vi "Begin.vi"() -> (0 "error out":errorcluster)   [LabVIEW 2013]
doc: "Called before other user functions, this VI is expected to open initial I/O refnums, load in file data, and do all program initialization. Notice that the <B>error out</B> terminal is simply used for data flow. Wiring it to other structures or subVIs ensures that this VI runs first."
uses:
  <vilib>/Rock Robotics/WPI/SafetyOutput/WPI_SafetyOutputConfigMenu.ctl
  <vilib>/Rock Robotics/WPI/DriverStation/WPI_DriverStationRobotMode2.ctl
  <vilib>/Rock Robotics/SystemInterfaces/DIO/FPGA_DIOPWMChannel.ctl
  <vilib>/Rock Robotics/SystemInterfaces/AI/FPGA_AIGyroChannel.ctl
  <vilib>/Rock Robotics/SystemInterfaces/Typedef/FPGA_TypedefAnalogModuleForGyro.ctl
  <vilib>/Rock Robotics/SystemInterfaces/DIO/FPGA_DIORelayChannel.ctl
  <vilib>/Rock Robotics/WPI/Joystick/WPI_JoystickDeviceEnum.ctl
  <vilib>/Rock Robotics/SystemInterfaces/DIO/FPGA_DIOChannel.ctl
  <vilib>/Rock Robotics/WPI/Encoder/WPI_EncoderType.ctl
  <vilib>/Rock Robotics/WPI/Relay/WPI_RelayDirection.ctl
  <vilib>/Rock Robotics/SystemInterfaces/Typedef/FPGA_TypedefDigitalModule.ctl
  <vilib>/Rock Robotics/WPI/Relay/WPI_RelayValue.ctl
  Robot Global Data.vi
  <vilib>/Rock Robotics/WPI/Counter/WPI_CounterDigitalInputToDigitalSource.vi
  <vilib>/Rock Robotics/WPI/MotorControl/WPI_MotorControlOpen Victor.vi
  <vilib>/Rock Robotics/WPI/RobotDrive/WPI_RobotDriveOpen4MotorWithVictor.vi
  <vilib>/Rock Robotics/WPI/Compressor/WPI_CompressorGetSetRefNum.vi
panel:
  out "error out 7":errorcluster
  out "error out 6":errorcluster
  out "error out 5":errorcluster
  out "error out 4":errorcluster
  out "error out 3":errorcluster
  out "error out 2":errorcluster
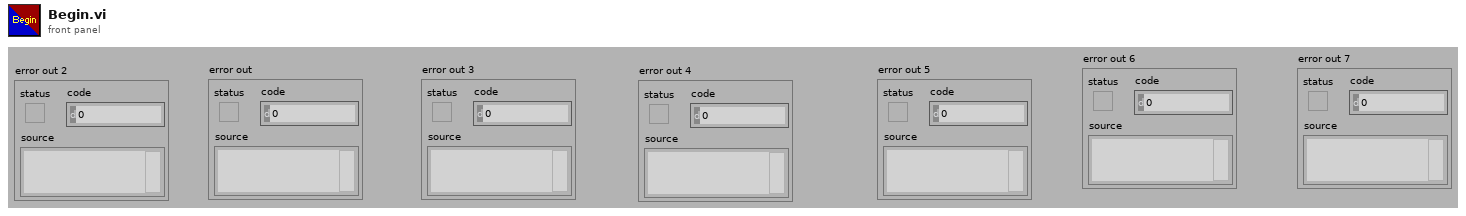
[diagram p1: front panel]
types:
  T1 = typedef "FPGA_DIOPWMChannel.ctl" = enum8{"PWM 1", "PWM 2", "PWM 3", "PWM 4", "PWM 5", "PWM 6", "PWM 7", "PWM 8", "PWM 9", "PWM 10", "Invalid"}
  T2 = typedef "WPI_RelayValue.ctl" = enum16{"Off", "On", "Forward", "Reverse"}
  T3 = typedef "FPGA_TypedefDigitalModule.ctl" = enum16{"Digital Module 1", "Digital Module 2"}
  T4 = typedef "FPGA_DIOChannel.ctl" = enum8{"DIO 1", "DIO 2", "DIO 3", "DIO 4", "DIO 5", "DIO 6", "DIO 7", "DIO 8", "DIO 9", "DIO 10", "DIO 11", "DIO 12", "DIO 13", "DIO 14", "Invalid"}
  T5 = typedef "FPGA_DIORelayChannel.ctl" = enum8{"Relay 1", "Relay 2", "Relay 3", "Relay 4", "Relay 5", "Relay 6", "Relay 7", "Relay 8", "Invalid"}
  T6 = typedef "WPI_RelayDirection.ctl" = enum16{"Both directions", "Forward only", "Reverse only"}
  T7 = typedef "WPI_EncoderType.ctl" = enum16{"1x", "2x", "4x"}
  T8 = typedef "WPI_JoystickDeviceEnum.ctl" = enum16{"USB 1", "USB 2", "USB 3", "USB 4", "Kinect 1", "Kinect 2"}
  T9 = typedef "FPGA_TypedefAnalogModuleForGyro.ctl" = enum16{"Analog Module 1"}
  T10 = typedef "FPGA_AIGyroChannel.ctl" = enum8{"AI 1", "AI 2", "Invalid"}
  T11 = typedef "WPI_DriverStationRobotMode2.ctl" = enum16{"Autonomous Disabled", "Autonomous Enabled", "Teleop Disabled", "Teleop Enabled", "Timeout", "Finish", "Test Disabled", "Test Enabled"}
  T12 = typedef "WPI_SafetyOutputConfigMenu.ctl" = enum16{"Enable", "Disable"}
  T13 = typedef "WPI_DigitalInputDevRef.ctl" = cluster{"DevStatus":errorcluster, "DIO Channel":T4, "Digital Module":T3}
  T14 = typedef "WPI_JoystickDevRef.ctl" = cluster{"Device":T8}
  T15 = typedef "WPI_MotorControlDeviceRef.ctl" = cluster{"DeviceStatus":errorcluster, "Type":enum16{"PWM", "CAN"}, "PWM":cluster{"Digital Module":T3, "PWM Channel":T1, "DeadBand":T16}, "CAN":cluster{"Device Number":u8, "Control Mode":T17, "Semaphore":T18, "Max Vout":dbl}, "Invert":bool, "TransformRef":T19, "InvTransformRef":T19}
  T16 = typedef "WPI_PWMDeadband.ctl" = cluster{"Name":string, "maxPositivePwm":i32, "minPositivePwm":i32, "centerPwm":i32, "maxNegativePwm":i32, "minNegativePwm":i32, "angularRange":u16}
  T17 = typedef "WPI_CANJaguar_ControlMode.ctl" = enum8{"Percent VBus", "Current", "Speed", "Position", "Voltage"}
  T18 = typedef "Semaphore RefNum" = refnum<k1>
  T19 = typedef "WPI_PWMTransform_ConPane.ctl" = refnum<vi>
  T20 = typedef "WPI_RelayDevRef.ctl" = cluster{"DevStatus":errorcluster, "Relay Channel":T5, "Digital Module":T3, "Relay Direction":T6}
  T21 = typedef "FPGA_CounterEncoderSourceConvertionLVSourceType.ctl" = cluster{"DevStatus":errorcluster, "AnalogTriggerMode?":bool, "DigitalMode":cluster{"Digital Module":T3, "DIO Channel":T22}, "AnalogTriggerMode":cluster{"AnalogTriggerIndex":T23, "OutputType":T24}}
  T22 = typedef "FPGA_DIODigitalSourceChannel.ctl" = enum8{"DIO 1", "DIO 2", "DIO 3", "DIO 4", "DIO 5", "DIO 6", "DIO 7", "DIO 8", "DIO 9", "DIO 10", "DIO 11", "DIO 12", "DIO 13", "DIO 14", "Disabled"}
  T23 = typedef "FPGA_AnalogTriggerIndex.ctl" = enum8{"Trig 0", "Trig 1", "Trig 2", "Trig 3", "Trig 4", "Trig 5", "Trig 6", "Trig 7", "Invalid"}
  T24 = typedef "FPGA_AnalogTriggerOutType.ctl" = enum16{"InWindow", "TriggerState", "Rising", "Falling"}
  T25 = typedef "WPI_RobotDriveDevRef.ctl" = cluster{"DevStatus":errorcluster, "Motors[]":T15[], "Square Inputs":bool, "Max Output":dbl, "Isochronous":bool}
  T26 = typedef "WPI_CompressorDevRef.ctl" = cluster{"DevStatus":errorcluster, "DigitalInputDevRef":T13, "RelayDevRef":T20}
  T27 = typedef "WPI_GyroDevRef.ctl" = cluster{"DevStatus":errorcluster, "Analog Module":T28, "Analog Channel":T29, "Offset":dbl, "Gain (VoltsPerDegree/Second)":dbl}
  T28 = typedef "FPGA_TypedefAnalogModule.ctl" = enum16{"Analog Module 1", "Analog Module 2"}
  T29 = typedef "FPGA_AIChannel.ctl" = enum8{"AI 1", "AI 2", "AI 3", "AI 4", "AI 5", "AI 6", "AI 7", "AI 8", "Invalid"}
  T30 = typedef "WPI_EncoderDevRef.ctl" = cluster{"DevStatus":errorcluster, "EncoderIndex":T31, "CounterIndex":T32, "DistancePerCount":dbl, "Decoding Type":T7}
  T31 = typedef "FPGA_EncoderIdx.ctl" = enum8{"Enc 0", "Enc 1", "Enc 2", "Enc 3", "Invalid"}
  T32 = typedef "FPGA_CounterCtrSystemIndex.ctl" = enum8{"Ctr 0", "Ctr 1", "Ctr 2", "Ctr 3", "Ctr 4", "Ctr 5", "Ctr 6", "Ctr 7", "Invalid"}
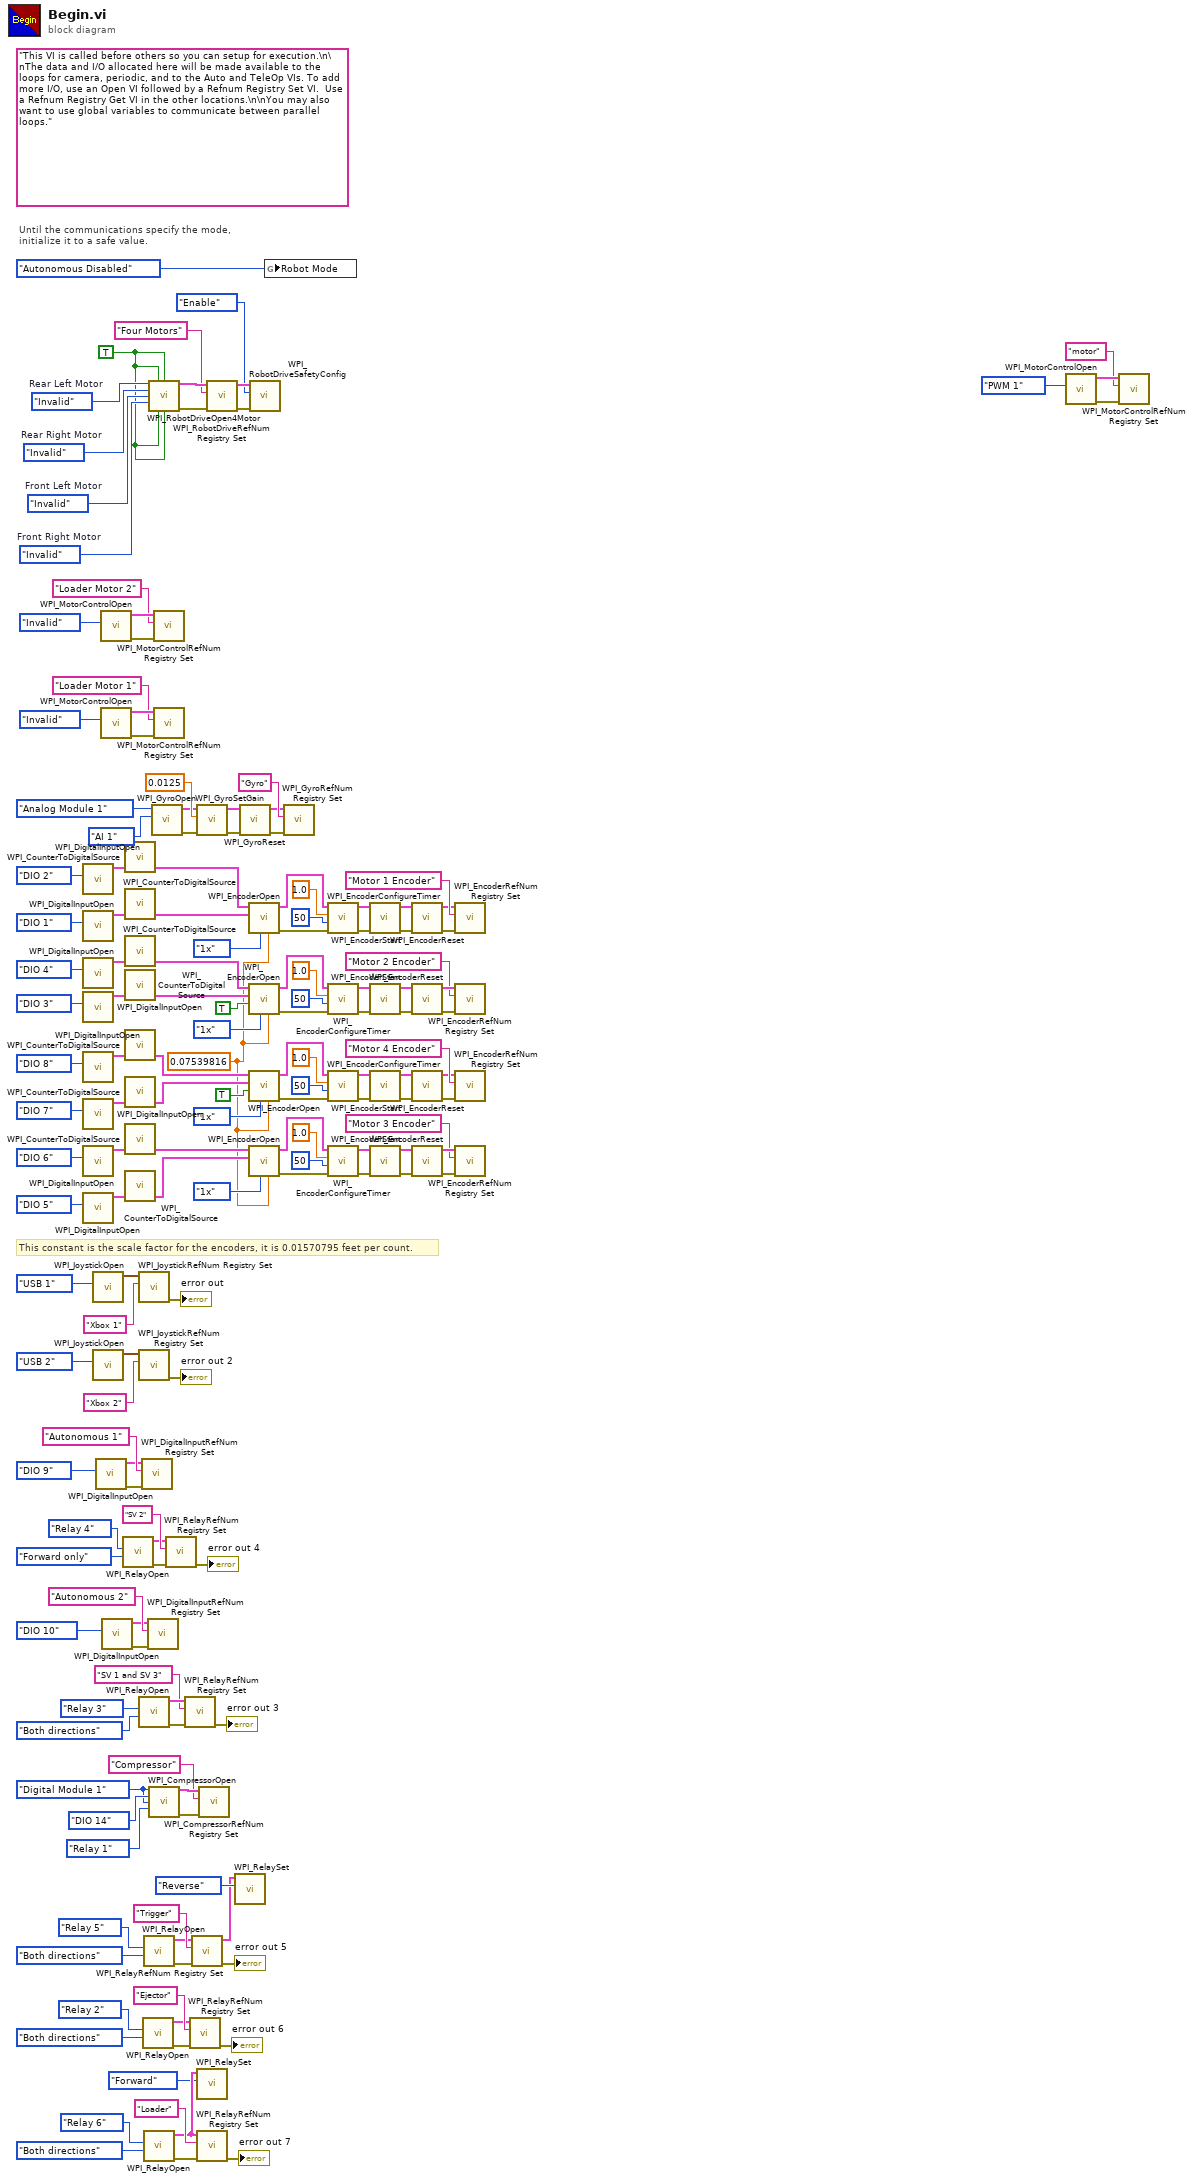
[diagram p0: block diagram]
diagram:
  w15 = FPGA_TypedefDigitalModule."Digital Module 1" ("Pressure Switch Digital Module (Module 1)")
  w5 = TRUE
  w6 = 0.07539816 ("DistancePerCount")
  w155 = FPGA_DIOPWMChannel."Invalid"  # Front Right Motor
  w156 = FPGA_DIOPWMChannel."Invalid"  # Front Left Motor
  w157 = FPGA_DIOPWMChannel."Invalid"  # Rear Right Motor
  w158 = FPGA_DIOPWMChannel."Invalid"  # Rear Left Motor
  (unwired) "This VI is called before others so you can setup for execution.\n\nThe data and I/O allocated here will be made available to the loops for camera, periodic, and to the Auto and TeleOp VIs. To add more I/O, use an Open VI followed by a Refnum Registry Set VI.  Use a Refnum Registry Get VI in the other locations.\n\nYou may also want to use global variables to communicate between parallel loops."
  # "This constant is the scale factor for the encoders, it is 0.01570795 feet per count."
  # "Until the communications specify the mode,\ninitialize it to a safe value."
  n1 = call <vilib>:"WPI_DigitalInputOpen.vi"("DIO Channel"=FPGA_DIOChannel."DIO 2") -> ("DigitalInputDevRef"=w62:T13)  [unwired: 2 in, 8 out]
  n2 = call <vilib>:"WPI_DigitalInputOpen.vi"("DIO Channel"=FPGA_DIOChannel."DIO 1") -> ("DigitalInputDevRef"=w61:T13)  [unwired: 2 in, 8 out]
  n3 = call <vilib>:"WPI_DigitalInputOpen.vi"("DIO Channel"=FPGA_DIOChannel."DIO 4") -> ("DigitalInputDevRef"=w93:T13)  [unwired: 2 in, 8 out]
  n4 = call <vilib>:"WPI_DigitalInputOpen.vi"("DIO Channel"=FPGA_DIOChannel."DIO 3") -> ("DigitalInputDevRef"=w94:T13)  [unwired: 2 in, 8 out]
  n5 = call <vilib>:"WPI_DigitalInputOpen.vi"("DIO Channel"=FPGA_DIOChannel."DIO 8") -> ("DigitalInputDevRef"=w98:T13)  [unwired: 2 in, 8 out]
  n6 = call <vilib>:"WPI_DigitalInputOpen.vi"("DIO Channel"=FPGA_DIOChannel."DIO 7") -> ("DigitalInputDevRef"=w97:T13)  [unwired: 2 in, 8 out]
  n7 = call <vilib>:"WPI_DigitalInputOpen.vi"("DIO Channel"=FPGA_DIOChannel."DIO 6") -> ("DigitalInputDevRef"=w130:T13)  [unwired: 2 in, 8 out]
  n8 = call <vilib>:"WPI_DigitalInputOpen.vi"("DIO Channel"=FPGA_DIOChannel."DIO 5") -> ("DigitalInputDevRef"=w131:T13)  [unwired: 2 in, 8 out]
  n9 = call <vilib>:"WPI_JoystickOpen.vi"("JoystickDevice"=WPI_JoystickDeviceEnum."USB 1") -> ("JoystickDevRef"=w57:T14)  [unwired: 10 in]
  n10 = call <vilib>:"WPI_JoystickOpen.vi"("JoystickDevice"=WPI_JoystickDeviceEnum."USB 2") -> ("JoystickDevRef"=w136:T14)  [unwired: 10 in]
  n11 = call <vilib>:"WPI_DigitalInputOpen.vi"("DIO Channel"=FPGA_DIOChannel."DIO 9") -> ("error out"=w27:errorcluster, "DigitalInputDevRef"=w29:T13)  [unwired: 2 in, 7 out]
  n12 = call-poly <vilib>:"WPI_MotorControlOpen.vi"("PWM Channel"=FPGA_DIOPWMChannel."Invalid") -> ("error out"=w20:errorcluster, "MotorControlDeviceRef"=w21:T15)  [unwired: 9 in]
  n13 = call-poly <vilib>:"WPI_MotorControlOpen.vi"("PWM Channel"=FPGA_DIOPWMChannel."Invalid") -> ("error out"=w22:errorcluster, "MotorControlDeviceRef"=w23:T15)  [unwired: 9 in]
  n14 = call <vilib>:"WPI_DigitalInputOpen.vi"("DIO Channel"=FPGA_DIOChannel."DIO 10") -> ("error out"=w26:errorcluster, "DigitalInputDevRef"=w28:T13)  [unwired: 2 in, 7 out]
  n15 = call <vilib>:"WPI_RelayOpen.vi"("Relay Direction"=WPI_RelayDirection."Forward only", "Relay Channel"=FPGA_DIORelayChannel."Relay 4") -> ("error out"=w50:errorcluster, "RelayDevRef"=w51:T20)  [unwired: 8 in]
  n16 = call-poly <vilib>:"WPI_CounterToDigitalSource.vi"("DigitalInputDevRef"=w62) -> ("Digital Source"=w63:T21)  [unwired: 6 out]
  n17 = call-poly <vilib>:"WPI_CounterToDigitalSource.vi"("DigitalInputDevRef"=w61) -> ("Digital Source"=w60:T21)  [unwired: 6 out]
  n18 = call-poly <vilib>:"WPI_CounterToDigitalSource.vi"("DigitalInputDevRef"=w93) -> ("Digital Source"=w92:T21)  [unwired: 6 out]
  n19 = call-poly <vilib>:"WPI_CounterToDigitalSource.vi"("DigitalInputDevRef"=w94) -> ("Digital Source"=w95:T21)  [unwired: 6 out]
  n20 = call-poly <vilib>:"WPI_CounterToDigitalSource.vi"("DigitalInputDevRef"=w98) -> ("Digital Source"=w99:T21)  [unwired: 6 out]
  n21 = call-poly <vilib>:"WPI_CounterToDigitalSource.vi"("DigitalInputDevRef"=w97) -> ("Digital Source"=w96:T21)  [unwired: 6 out]
  n22 = call-poly <vilib>:"WPI_CounterToDigitalSource.vi"("DigitalInputDevRef"=w130) -> ("Digital Source"=w129:T21)  [unwired: 6 out]
  n23 = call-poly <vilib>:"WPI_CounterToDigitalSource.vi"("DigitalInputDevRef"=w131) -> ("Digital Source"=w132:T21)  [unwired: 6 out]
  n24 = call <vilib>:"WPI_JoystickRefNum Registry Set.vi"("refnum name"="Xbox 1", "JoystickDevRef"=w57) -> ("error out"=→"error out":errorcluster)  [unwired: 8 in, 1 out]
  n25 = call <vilib>:"WPI_JoystickRefNum Registry Set.vi"("refnum name"="Xbox 2", "JoystickDevRef"=w136) -> ("error out"=→"error out 2":errorcluster)  [unwired: 8 in, 1 out]
  n26 = call <vilib>:"WPI_RelayOpen.vi"("Relay Direction"=WPI_RelayDirection."Both directions", "Relay Channel"=FPGA_DIORelayChannel."Relay 3") -> ("error out"=w143:errorcluster, "RelayDevRef"=w142:T20)  [unwired: 8 in]
  n27 = call <vilib>:"WPI_DigitalInputRefNum Registry Set.vi"("error in (no error)"=w27, "refnum name"="Autonomous 1", "DigitalInputDevRef"=w29) -> ()  [unwired: 7 in, 2 out]
  n28 = call <vilib>:"WPI_RelayOpen.vi"("Relay Direction"=WPI_RelayDirection."Both directions", "Relay Channel"=FPGA_DIORelayChannel."Relay 2") -> ("error out"=w39:errorcluster, "RelayDevRef"=w40:T20)  [unwired: 8 in]
  n29 = call <vilib>:"WPI_RelayOpen.vi"("Relay Direction"=WPI_RelayDirection."Both directions", "Relay Channel"=FPGA_DIORelayChannel."Relay 5") -> ("error out"=w49:errorcluster, "RelayDevRef"=w10:T20)  [unwired: 8 in]
  n30 = call <vilib>:"WPI_RelayOpen.vi"("Relay Direction"=WPI_RelayDirection."Both directions", "Relay Channel"=FPGA_DIORelayChannel."Relay 6") -> ("error out"=w38:errorcluster, "RelayDevRef"=w8:T20)  [unwired: 8 in]
  n31 = call <vilib>:"WPI_DigitalInputRefNum Registry Set.vi"("error in (no error)"=w26, "refnum name"="Autonomous 2", "DigitalInputDevRef"=w28) -> ()  [unwired: 7 in, 2 out]
  n32 = call-poly <vilib>:"WPI_RobotDriveOpen4Motor.vi"("Rear Left Motor"=w158, "Rear Left Motor Inverted"=w5, "Rear Right Motor Inverted"=w5, "Rear Right Motor"=w157, "Front Left Motor"=w156, "Front Right Motor"=w155, "Front Left Motor Inverted"=w5, "Front Right Motor Inverted"=w5) -> ("RobotDriveDevRef"=w164:T25, "error out"=w162:errorcluster)  [unwired: 6 in]
  n33 = call <vilib>:"WPI_CompressorOpen.vi"("Pressure Switch Digital Module (Module 1)"=w15, "Pressure Switch DIO Channel"=FPGA_DIOChannel."DIO 14", "Relay Digital Module (Module 1)"=w15, "Relay Channel"=FPGA_DIORelayChannel."Relay 1") -> ("CompressorDevRef"=w13:T26, "error out"=w14:errorcluster)  [unwired: 10 in]
  n34 = call <vilib>:"WPI_GyroOpen.vi"("Analog Channel"=FPGA_AIGyroChannel."AI 1" ("Channel"), "Analog Module (Module 1)"=FPGA_TypedefAnalogModuleForGyro."Analog Module 1" ("Analog Module")) -> ("error out"=w149:errorcluster, "GyroDevRef"=w150:T27)  [unwired: 4 in, 4 out]
  n35 = call <vilib>:"WPI_MotorControlRefNum Registry Set.vi"("error in (no error)"=w20, "refnum name"="Loader Motor 2", "MotorControlDevRef"=w21) -> ()  [unwired: 7 in, 2 out]
  n36 = call <vilib>:"WPI_MotorControlRefNum Registry Set.vi"("error in (no error)"=w22, "refnum name"="Loader Motor 1", "MotorControlDevRef"=w23) -> ()  [unwired: 7 in, 2 out]
  n37 = call <vilib>:"WPI_RelayRefNum Registry Set.vi"("error in (no error)"=w50, "refnum name"="SV 2", "RelayDevRef"=w51) -> ("error out"=→"error out 4":errorcluster)  [unwired: 7 in, 1 out]
  n38 = call <vilib>:"WPI_RelayRefNum Registry Set.vi"("error in (no error)"=w143, "refnum name"="SV 1 and SV 3", "RelayDevRef"=w142) -> ("error out"=→"error out 3":errorcluster)  [unwired: 7 in, 1 out]
  n39 = call <vilib>:"WPI_RelayRefNum Registry Set.vi"("error in (no error)"=w39, "refnum name"="Ejector", "RelayDevRef"=w40) -> ("error out"=→"error out 6":errorcluster)  [unwired: 7 in, 1 out]
  n40 = call <vilib>:"WPI_RelayRefNum Registry Set.vi"("error in (no error)"=w49, "refnum name"="Trigger", "RelayDevRef"=w10) -> ("error out"=→"error out 5":errorcluster, "RelayDevRef"=w9:T20)  [unwired: 7 in]
  n41 = call <vilib>:"WPI_GyroSetGain.vi"("error in (no error)"=w149, "Gain (VoltsPerDegree/Second)"=0.0125, "GyroDevRef"=w150) -> ("error out"=w147:errorcluster, "GyroDevRef"=w148:T27)  [unwired: 7 out]
  n42 = call <vilib>:"WPI_RelaySet.vi"("RelayValue"=WPI_RelayValue."Forward", "RelayDevRef"=w8) -> ()  [unwired: 8 in, 2 out]
  n43 = call <vilib>:"WPI_RelayRefNum Registry Set.vi"("error in (no error)"=w38, "refnum name"="Loader", "RelayDevRef"=w8) -> ("error out"=→"error out 7":errorcluster)  [unwired: 7 in, 1 out]
  n44 = call <vilib>:"WPI_CompressorRefNum Registry Set.vi"("error in (no error)"=w14, "refnum name"="Compressor", "CompressorDevRef"=w13) -> ()  [unwired: 7 in, 2 out]
  n45 = call <vilib>:"WPI_RobotDriveRefNum Registry Set.vi"("error in (no error)"=w162, "refnum name"="Four Motors", "RobotDriveDevRef"=w164) -> ("error out"=w144:errorcluster, "RobotDriveDevRef"=w161:T25)  [unwired: 7 out]
  n46 = call <vilib>:"WPI_RelaySet.vi"("RelayValue"=WPI_RelayValue."Reverse", "RelayDevRef"=w9) -> ()  [unwired: 8 in, 2 out]
  n47 = call <vilib>:"WPI_GyroReset.vi"("error in (no error)"=w147, "GyroDevRef"=w148) -> ("error out"=w145:errorcluster, "GyroDevRef"=w146:T27)  [unwired: 8 out]
  n48 = call <vilib>:"WPI_EncoderOpen.vi"("DistancePerCount"=w6, "Decoding Type"=WPI_EncoderType."1x", "BSource"=w60, "ASource"=w63) -> ("error out"=w71:errorcluster, "EncoderDevRef"=w65:T30)  [unwired: 4 in, 2 out]
  n49 = call <vilib>:"WPI_EncoderOpen.vi"("DistancePerCount"=w6, "Decoding Type"=WPI_EncoderType."1x", "Invert Direction (False)"=TRUE, "BSource"=w95, "ASource"=w92) -> ("error out"=w84:errorcluster, "EncoderDevRef"=w90:T30)  [unwired: 3 in, 2 out]
  n50 = call <vilib>:"WPI_EncoderOpen.vi"("DistancePerCount"=w6, "Decoding Type"=WPI_EncoderType."1x", "Invert Direction (False)"=TRUE, "BSource"=w96, "ASource"=w99) -> ("error out"=w107:errorcluster, "EncoderDevRef"=w101:T30)  [unwired: 3 in, 2 out]
  n51 = call <vilib>:"WPI_EncoderOpen.vi"("DistancePerCount"=w6, "Decoding Type"=WPI_EncoderType."1x", "BSource"=w132, "ASource"=w129) -> ("error out"=w121:errorcluster, "EncoderDevRef"=w127:T30)  [unwired: 4 in, 2 out]
  n52 = call <vilib>:"WPI_RobotDriveSafetyConfig.vi"("error in (no error)"=w144, "mode"=WPI_SafetyOutputConfigMenu."Enable", "RobotDriveDevRef"=w161) -> ()  [unwired: 7 in, 2 out]
  n53 = global write "Robot Global Data.vi" "Robot Mode"(WPI_DriverStationRobotMode2."Autonomous Disabled" ("Robot Mode")) -> ()
  n54 = call <vilib>:"WPI_GyroRefNum Registry Set.vi"("error in (no error)"=w145, "refnum name"="Gyro", "GyroDevRef"=w146) -> ()  [unwired: 7 in, 2 out]
  n55 = call <vilib>:"WPI_EncoderConfigureTimer.vi"("error in (no error)"=w71, "Number Samples to Average"=u8 50, "Minimum Rate"=1.0, "EncoderDevRef"=w65) -> ("error out"=w70:errorcluster, "EncoderDevRef"=w64:T30)  [unwired: 6 out]
  n56 = call <vilib>:"WPI_EncoderConfigureTimer.vi"("error in (no error)"=w84, "Number Samples to Average"=u8 50, "Minimum Rate"=1.0, "EncoderDevRef"=w90) -> ("error out"=w85:errorcluster, "EncoderDevRef"=w91:T30)  [unwired: 6 out]
  n57 = call <vilib>:"WPI_EncoderConfigureTimer.vi"("error in (no error)"=w107, "Number Samples to Average"=u8 50, "Minimum Rate"=1.0, "EncoderDevRef"=w101) -> ("error out"=w106:errorcluster, "EncoderDevRef"=w100:T30)  [unwired: 6 out]
  n58 = call <vilib>:"WPI_EncoderConfigureTimer.vi"("error in (no error)"=w121, "Number Samples to Average"=u8 50, "Minimum Rate"=1.0, "EncoderDevRef"=w127) -> ("error out"=w122:errorcluster, "EncoderDevRef"=w128:T30)  [unwired: 6 out]
  n59 = call <vilib>:"WPI_EncoderStart.vi"("error in (no error)"=w70, "EncoderDevRef"=w64) -> ("error out"=w69:errorcluster, "EncoderDevRef"=w68:T30)  [unwired: 8 out]
  n60 = call <vilib>:"WPI_EncoderStart.vi"("error in (no error)"=w85, "EncoderDevRef"=w91) -> ("error out"=w86:errorcluster, "EncoderDevRef"=w87:T30)  [unwired: 8 out]
  n61 = call <vilib>:"WPI_EncoderStart.vi"("error in (no error)"=w106, "EncoderDevRef"=w100) -> ("error out"=w105:errorcluster, "EncoderDevRef"=w104:T30)  [unwired: 8 out]
  n62 = call <vilib>:"WPI_EncoderStart.vi"("error in (no error)"=w122, "EncoderDevRef"=w128) -> ("error out"=w123:errorcluster, "EncoderDevRef"=w124:T30)  [unwired: 8 out]
  n63 = call <vilib>:"WPI_EncoderReset.vi"("error in (no error)"=w69, "EncoderDevRef"=w68) -> ("error out"=w72:errorcluster, "EncoderDevRef"=w73:T30)  [unwired: 8 out]
  n64 = call <vilib>:"WPI_EncoderReset.vi"("error in (no error)"=w86, "EncoderDevRef"=w87) -> ("error out"=w83:errorcluster, "EncoderDevRef"=w82:T30)  [unwired: 8 out]
  n65 = call <vilib>:"WPI_EncoderReset.vi"("error in (no error)"=w105, "EncoderDevRef"=w104) -> ("error out"=w108:errorcluster, "EncoderDevRef"=w109:T30)  [unwired: 8 out]
  n66 = call <vilib>:"WPI_EncoderReset.vi"("error in (no error)"=w123, "EncoderDevRef"=w124) -> ("error out"=w120:errorcluster, "EncoderDevRef"=w119:T30)  [unwired: 8 out]
  n67 = call <vilib>:"WPI_EncoderRefNum Registry Set.vi"("error in (no error)"=w72, "refnum name"="Motor 1 Encoder", "EncoderDevRef"=w73) -> ()  [unwired: 7 in, 2 out]
  n68 = call <vilib>:"WPI_EncoderRefNum Registry Set.vi"("error in (no error)"=w83, "refnum name"="Motor 2 Encoder", "EncoderDevRef"=w82) -> ()  [unwired: 7 in, 2 out]
  n69 = call <vilib>:"WPI_EncoderRefNum Registry Set.vi"("error in (no error)"=w108, "refnum name"="Motor 4 Encoder", "EncoderDevRef"=w109) -> ()  [unwired: 7 in, 2 out]
  n70 = call <vilib>:"WPI_EncoderRefNum Registry Set.vi"("error in (no error)"=w120, "refnum name"="Motor 3 Encoder", "EncoderDevRef"=w119) -> ()  [unwired: 7 in, 2 out]
  n71 = call-poly <vilib>:"WPI_MotorControlOpen.vi"("PWM Channel"=FPGA_DIOPWMChannel."PWM 1") -> ("error out"=w2:errorcluster, "MotorControlDeviceRef"=w3:T15)  [unwired: 9 in]
  n72 = call <vilib>:"WPI_MotorControlRefNum Registry Set.vi"("error in (no error)"=w2, "refnum name"="motor", "MotorControlDevRef"=w3) -> ()  [unwired: 7 in, 2 out]
